vi "STB-Top.vi"() -> ()   [LabVIEW 2024]
doc: "This template is for the Queued Message Handler design pattern.\n\nThe Event Handling Loop generates messages based on user interface actions.\n\nThe Message Handling Loop processes messages generated by the Event Handling Loop, or by other messages. The messages are string values, so new messages can be added easily to the Message Cases case structure in the Message Handling Loop. Each message cluster can also provide an optional value for Message Data, which is a variant that can be converted to whatever message-specific data is required."
uses:
  e6b95c05-a4c0-4812-af30-7667d0d88226.vi
  <resource>/objmgr/daqmx.rc
  <vilib>/Utility/miscctls.llb/LVRectTypeDef.ctl
  <vilib>/Utility/TDMS File Viewer/NI_TDMS File Viewer.lvlib
panel:
  in  "Logging":bool
  out "IsLogging?":bool
  in  "Stop Button":bool
  in  "Save Settings":bool
  in  "Tab Control":T1(tab)
  in  "NI9205_Ch_3":bool
  in  "NI9205_Ch_2":bool
  in  "NI9205_Ch_1":bool
  in  "NI9205_Ch_0":bool
  in  "NI9219_Ch_3":bool
  in  "NI9219_Ch_2":bool
  in  "NI9219_Ch_1":bool
  in  "NI9219_Ch_0":bool
  in  "NI9219_Ch_2_Strain Gauge":bool
  in  "NI9219_Ch_1_Strain Gauge":bool
  in  "NI9219_Ch_0_Strain Gauge":bool
  in  "NI9219_Ch_0_Load Cell":bool
  out "Warnings & Messages":string
  out "NI9219_Channel 0-2 Chart":dynamicdata(graph)
  out "Temperature_6":dbl caption="Strain_2"
  out "Temperature_5":dbl caption="Strain_1"
  out "Temperature_4":dbl caption="Strain_0"
  out "NI9219_Channel 0Chart":dynamicdata(graph)
  out "Temperature_0":dbl caption="Force_0"
  out "NI9219_Channel 0-3 Chart":dynamicdata(graph)
  out "Temperature_3":dbl caption="Strain_3"
  out "Temperature_2":dbl caption="Strain_2"
  out "Temperature_1":dbl caption="Strain_1"
  out "Temperature_0":dbl caption="Strain_0"
  out "NI9205_Channel 0-3 Chart":dynamicdata(graph)
  out "Current_3":dbl caption="Voltage_3"
  out "Current_2":dbl caption="Voltage_2"
  out "Current_1":dbl caption="Voltage_1"
  out "Current_0":dbl caption="Voltage_0"
  out "Select File Path Analysis":path caption="Select File Path"
  in  "Offline Analysis":bool
  out "TDMS File Path":path
  # "These controls have associated \"Value Changed\" events configured in the Event Structure on the diagram.\n\nReplace them (and reconfigure the Event Structure) with the controls you need for your application."
  # "This template is for the Queued Message Handler design pattern.\n\nSee the block diagram for more information on how to use this template."
  # "Slot 1:NI 9219"
  # "Slot 1:NI 9219"
  # "Slot 2:NI 9219"
  # "NI 9205"
  # "Warnings & Messages"
  # "Picture"
  # "Channel 0-2"
  # "Channel 0"
  # "Channel 0-3"
  # "Channel 0-3"
  # "Analysis"
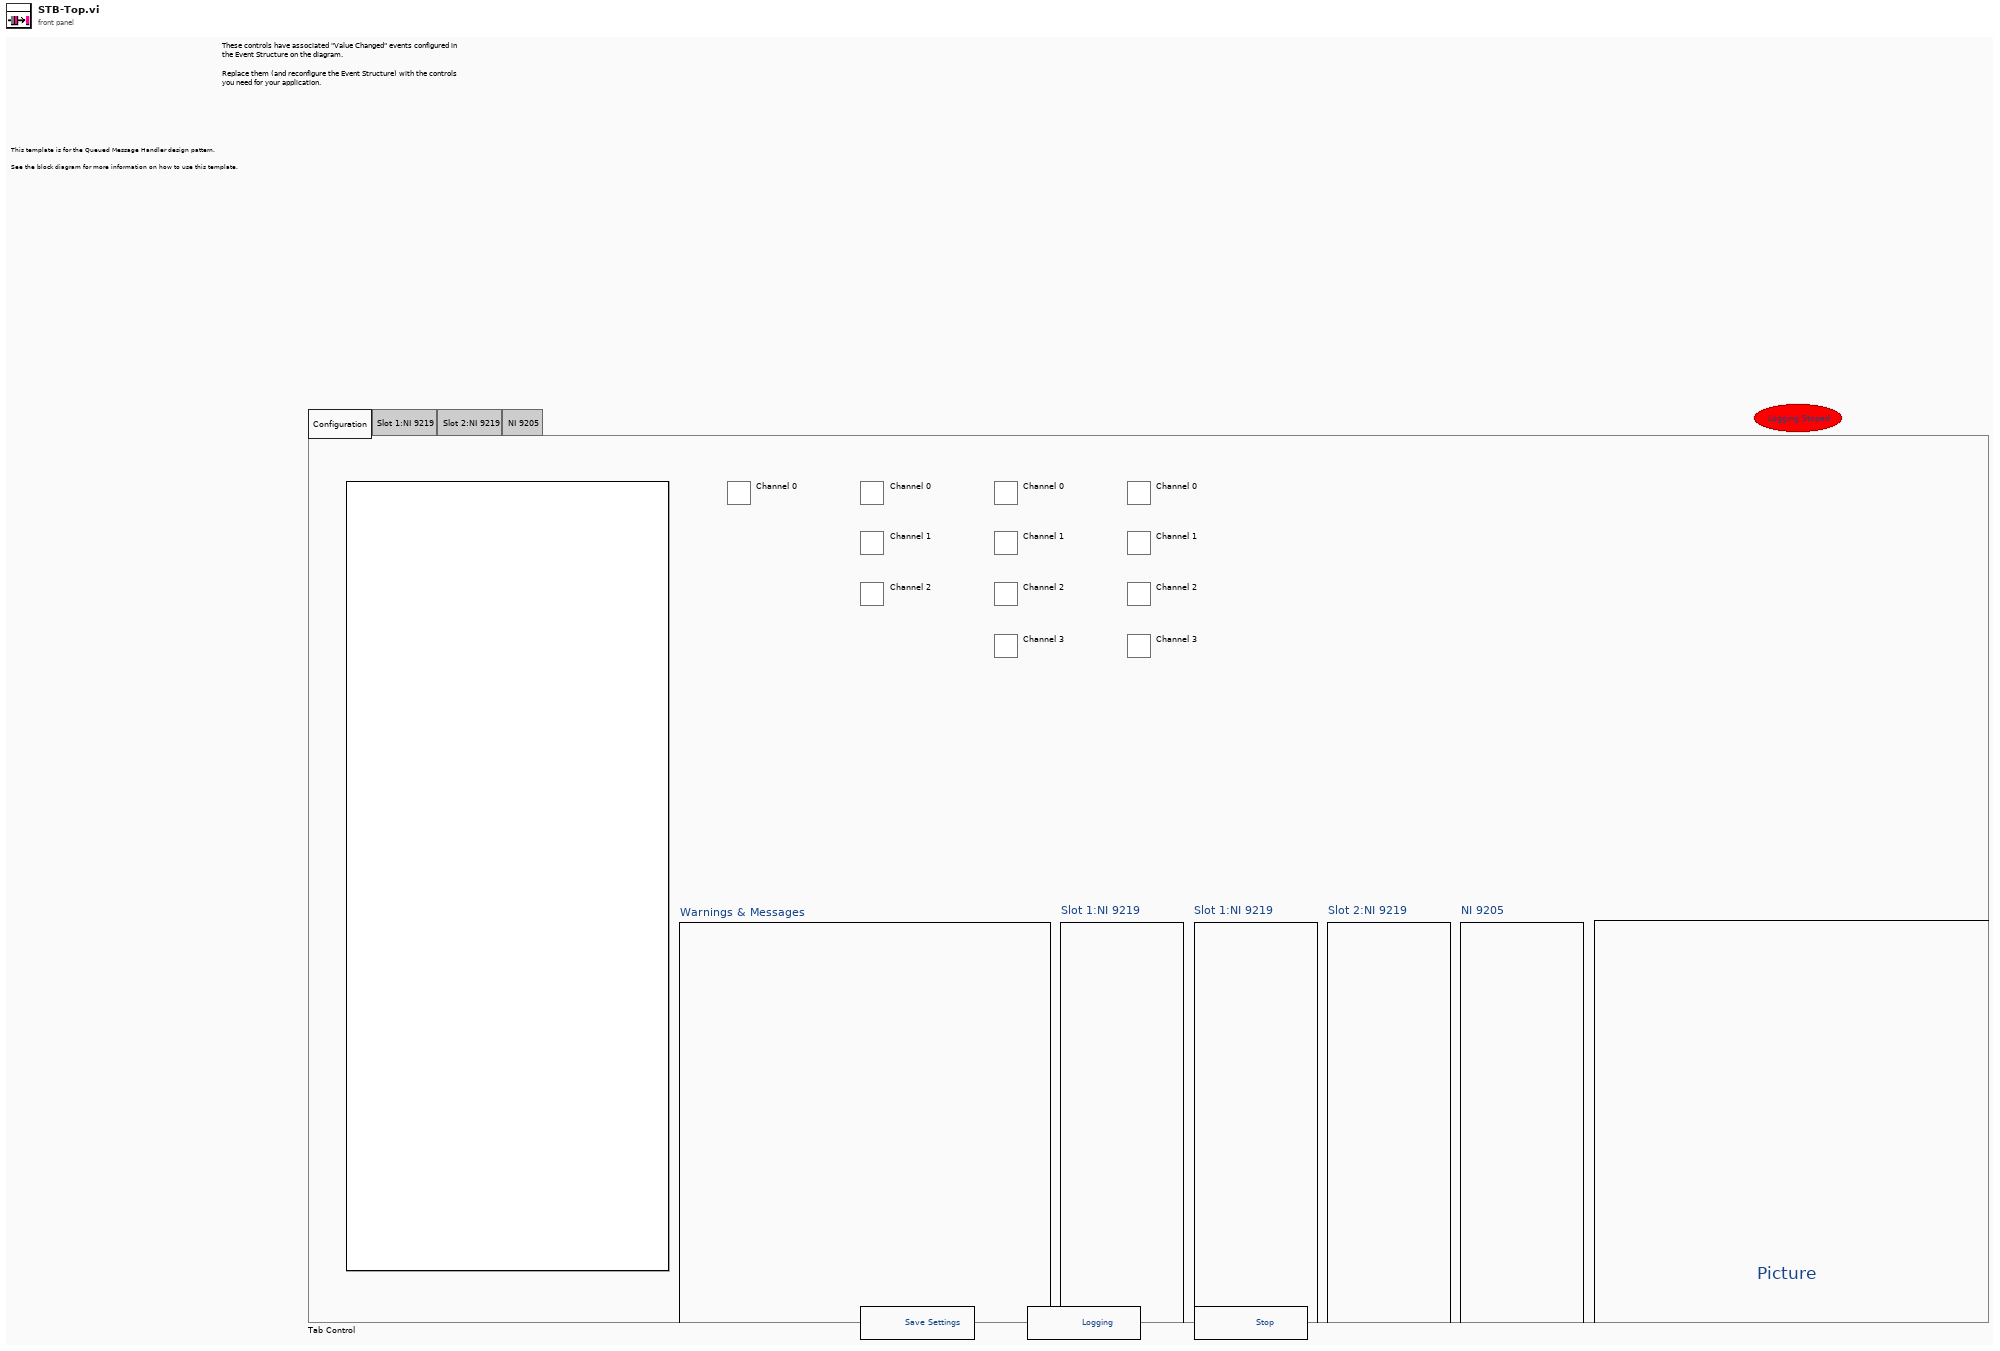
[diagram p1: front panel]
types:
  T1 = enum32{"Configuration", "Slot 1:NI 9219", "Slot 2:NI 9219", "NI 9205", "Offline Analysis"}
  T2 = typedef "LVRectTypeDef.ctl" = cluster{"Left":i16, "Top":i16, "Right":i16, "Bottom":i16}
  T3 = enum16{"open", "open or create", "create or replace", "create", "open (read-only)"}
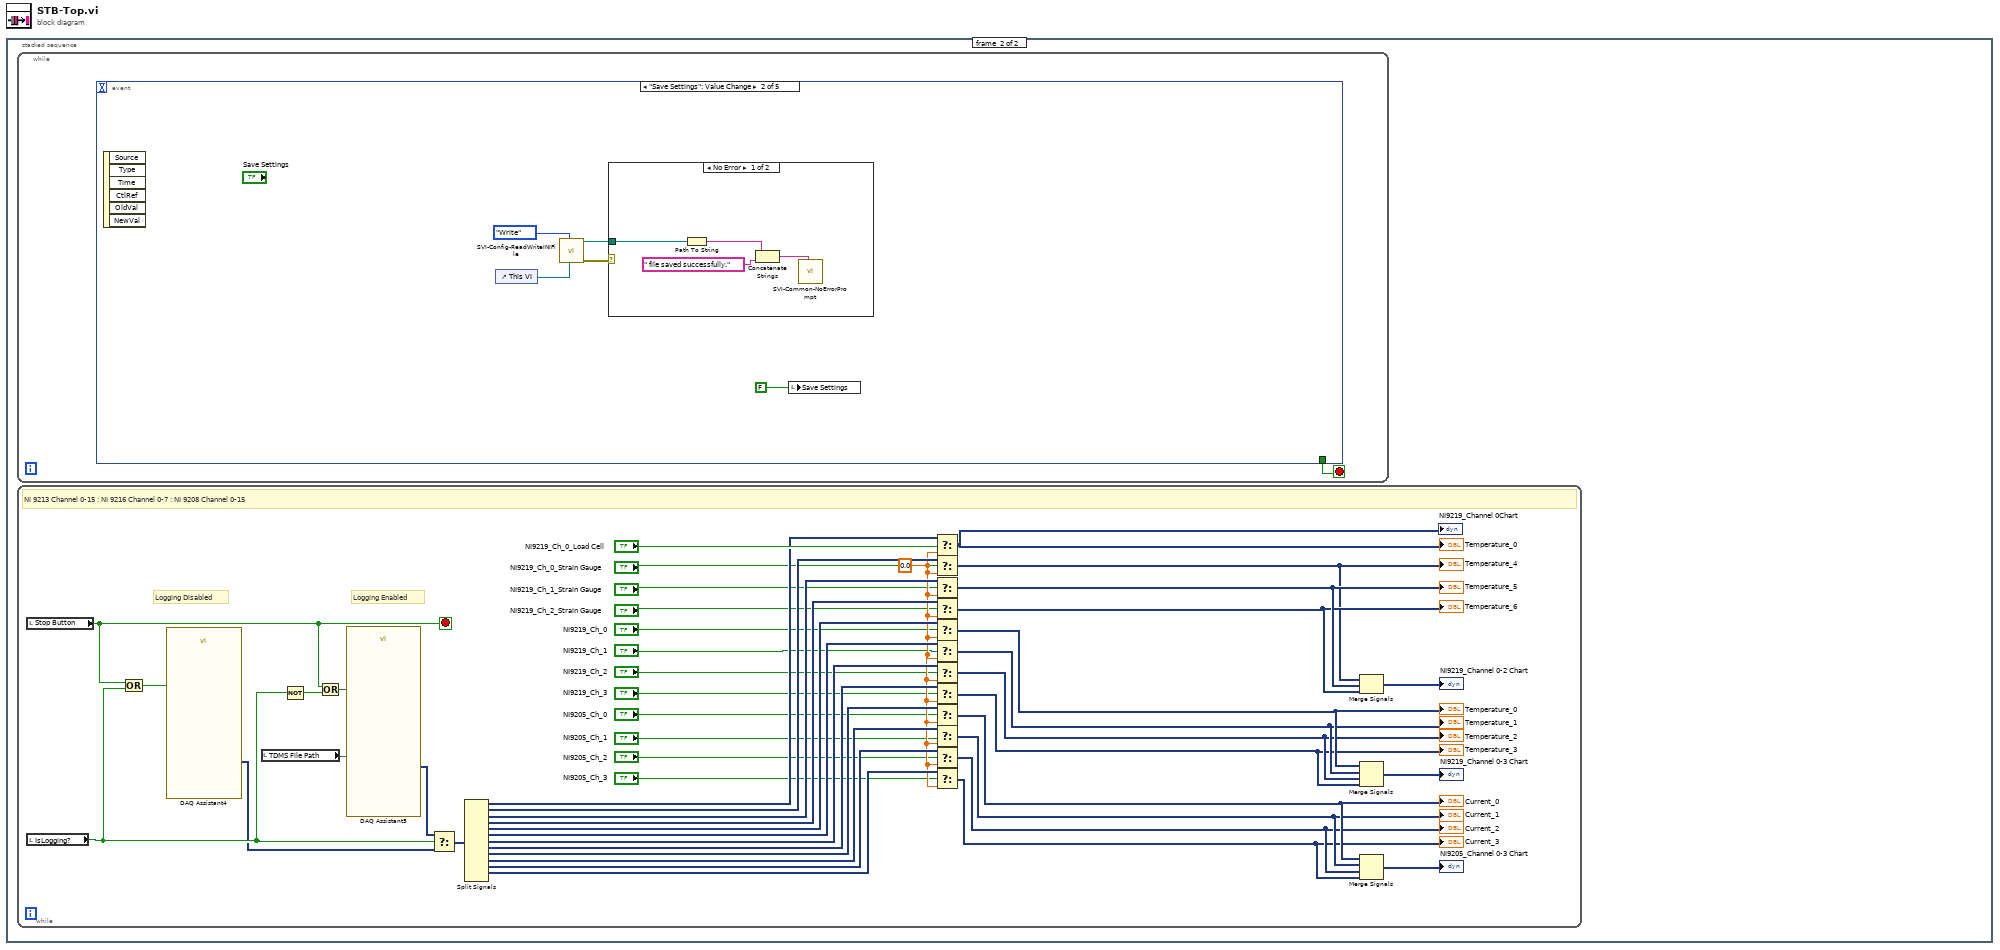
[diagram p0: block diagram]
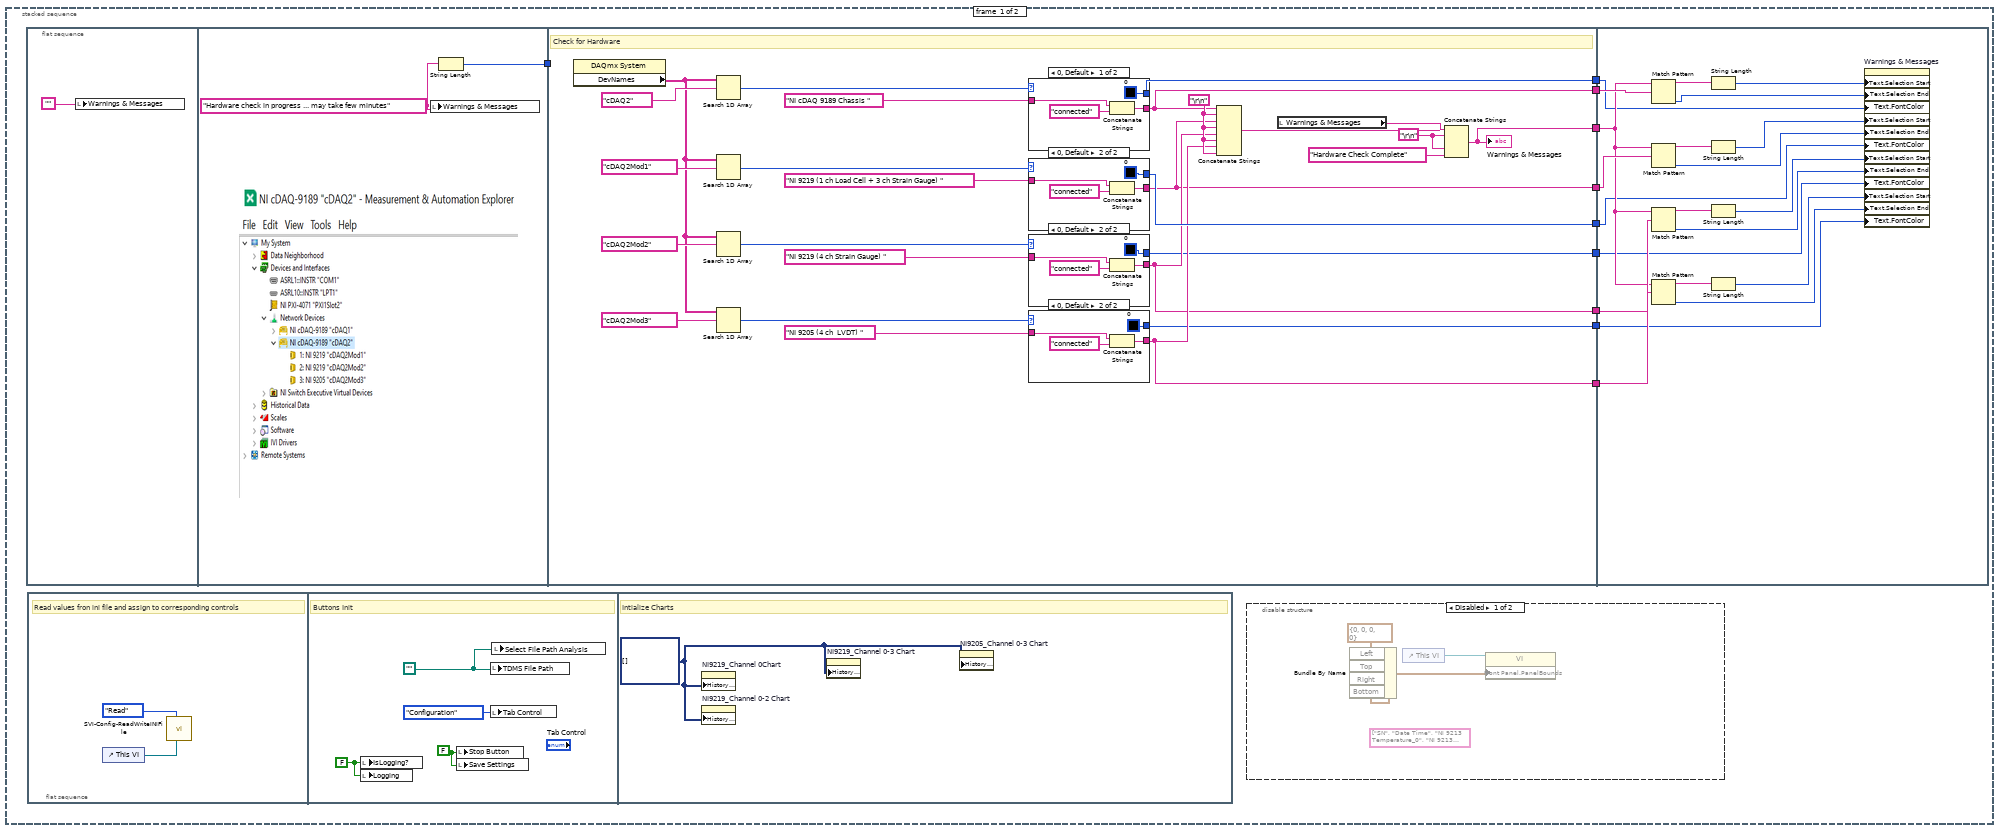
[diagram p2: hidden frame]
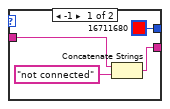
[diagram p4: hidden frame]
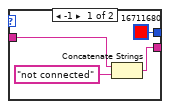
[diagram p5: hidden frame]
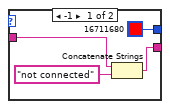
[diagram p6: hidden frame]
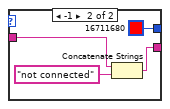
[diagram p7: hidden frame]
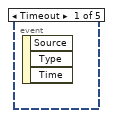
[diagram p8: hidden frame]
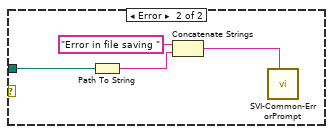
[diagram p9: hidden frame]
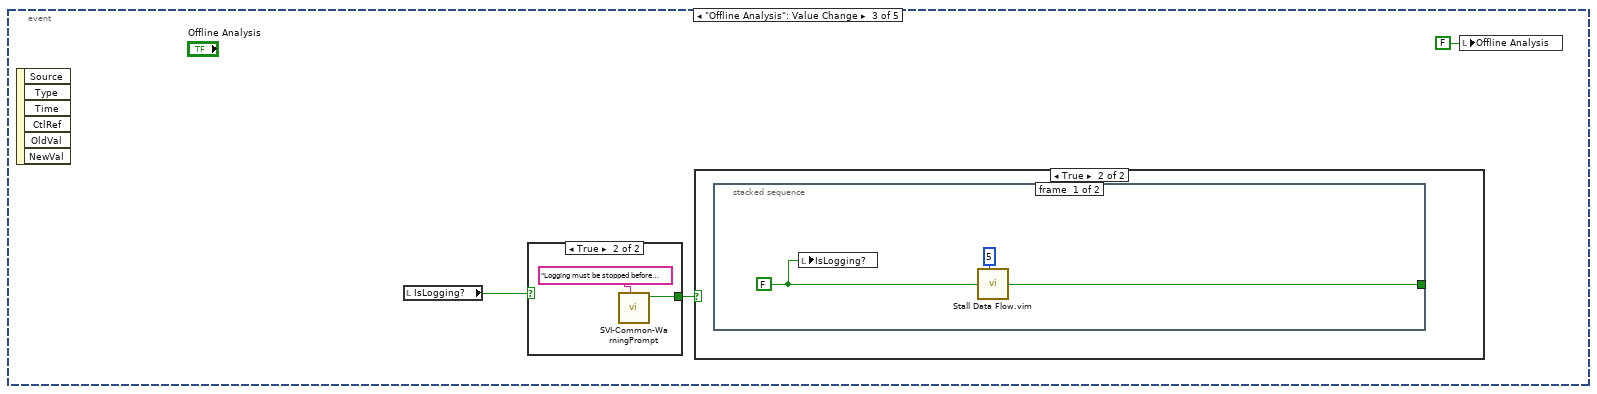
[diagram p10: hidden frame]
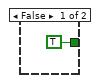
[diagram p11: hidden frame]
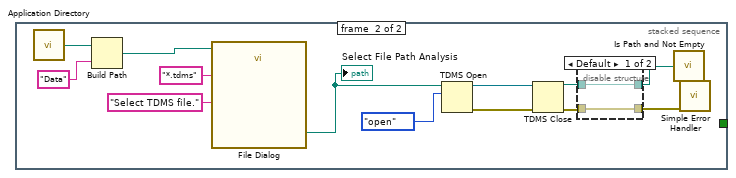
[diagram p13: hidden frame]
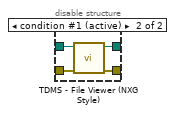
[diagram p14: hidden frame]
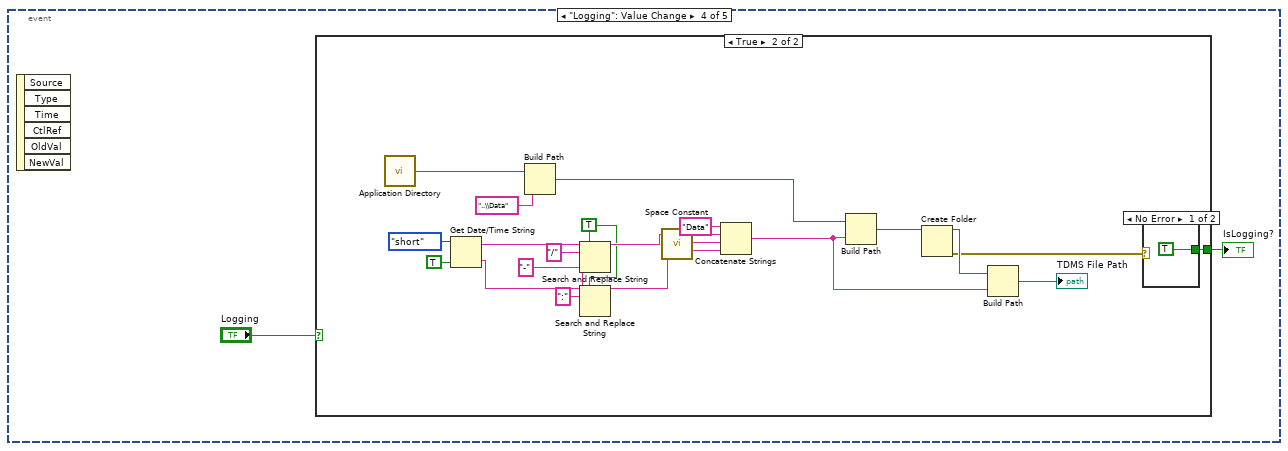
[diagram p15: hidden frame]
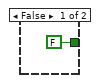
[diagram p16: hidden frame]
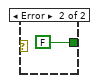
[diagram p17: hidden frame]
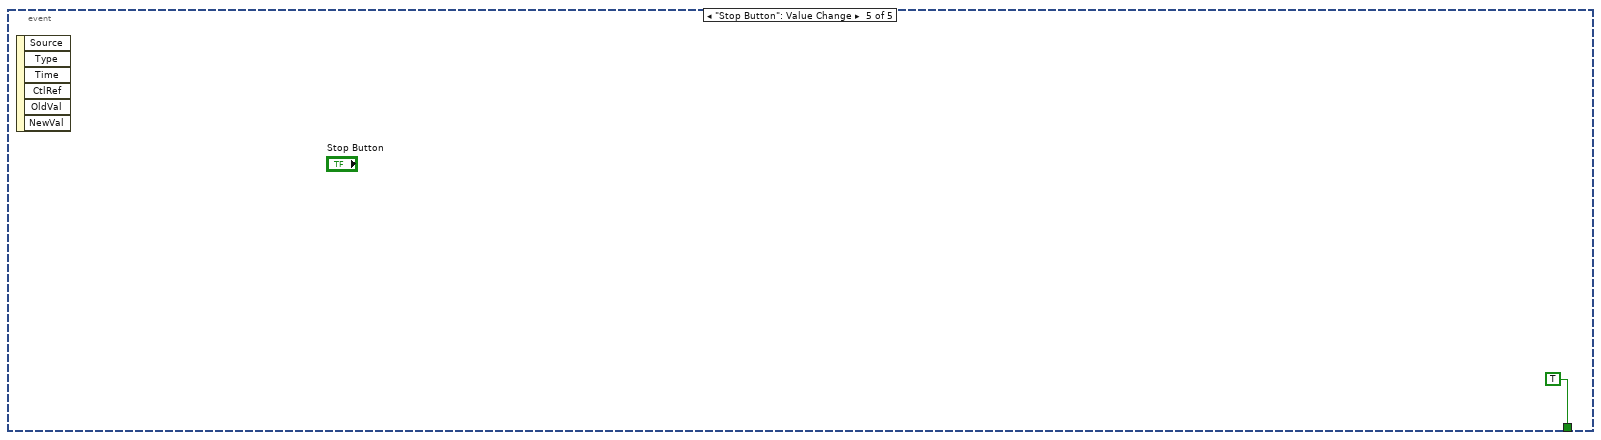
[diagram p18: hidden frame]
diagram:
  n1 = stacked-sequence {
    frame #0 {
      n2 = flat-sequence {
        tunnel: [w22] -> w10
        tunnel: w10 -> [_]
        tunnel: [w38] -> w9
        tunnel: [w37] -> w8
        tunnel: [w30] -> w7
        tunnel: [w29] -> w6
        tunnel: [w35] -> w5
        tunnel: [w34] -> w4
        tunnel: [w33] -> w3
        tunnel: [w32] -> w2
        tunnel: [w31] -> w1
        tunnel: w9 -> [w92]
        tunnel: w8 -> [w89]
        tunnel: w7 -> [w86]
        tunnel: w6 -> [w83]
        tunnel: w5 -> [w99]
        tunnel: w4 -> [w98]
        tunnel: w3 -> [w97]
        tunnel: w2 -> [w96]
        tunnel: w1 -> [w95]
        frame #0 {
          n3 = local write "Warnings & Messages"("") -> ()
        }
        frame #1 {
          w23 = "Hardware check in progress ... may take few minutes"
          n4 = local write "Warnings & Messages"(w23) -> ()
          n5 = String Length(string=w23) -> (length=w22:i32)
        }
        frame #2 {
          w40 = "\r\n"
          w47 = "\r\n"
          # "Check for Hardware"
          n6 = property class="DAQmx System"() -> ("DevNames"=w42:tag[])  [unwired: 2 in, 2 out]
          n7 = Search 1D Array(1D array=w42, element=tag "cDAQ2") -> (index of element=w28:i32)  [unwired: 1 in]
          n8 = Search 1D Array(1D array=w42, element=tag "cDAQ2Mod1") -> (index of element=w25:i32)  [unwired: 1 in]
          n9 = Search 1D Array(1D array=w42, element=tag "cDAQ2Mod2") -> (index of element=w24:i32)  [unwired: 1 in]
          n10 = Search 1D Array(1D array=w42, element=tag "cDAQ2Mod3") -> (index of element=w27:i32)  [unwired: 1 in]
          n11 = case shown="0, Default" w28 {
            tunnel: "NI cDAQ 9189 Chassis " -> [w78 w82]
            tunnel: [w76 w80] -> w32
            tunnel: [u32 0 ("Text.Text Colors:Text Color") u32 16711680 ("Text.Text Colors:Text Color")] -> w38
            frame 0, Default {
              n12 = Concatenate Strings(w78, "connected" ("string")) -> (w76:string)
            }
            frame -1 {
              n13 = Concatenate Strings(w82, "not connected" ("string")) -> (w80:string)
            }
          }
          n14 = case shown="0, Default" w25 {
            tunnel: "NI 9219 (1 ch Load Cell + 3 ch Strain Gauge) " -> [w70 w74]
            tunnel: [w68 w72] -> w33
            tunnel: [u32 16711680 ("Text.Text Colors:Text Color") u32 0 ("Text.Text Colors:Text Color")] -> w37
            frame -1 {
              n15 = Concatenate Strings(w70, "not connected" ("string")) -> (w68:string)
            }
            frame 0, Default {
              n16 = Concatenate Strings(w74, "connected" ("string")) -> (w72:string)
            }
          }
          n17 = case shown="0, Default" w24 {
            tunnel: "NI 9219 (4 ch Strain Gauge) " -> [w62 w66]
            tunnel: [w60 w64] -> w34
            tunnel: [u32 16711680 ("Text.Text Colors:Text Color") u32 0 ("Text.Text Colors:Text Color")] -> w30
            frame -1 {
              n18 = Concatenate Strings(w62, "not connected" ("string")) -> (w60:string)
            }
            frame 0, Default {
              n19 = Concatenate Strings(w66, "connected" ("string")) -> (w64:string)
            }
          }
          n20 = case shown="0, Default" w27 {
            tunnel: "NI 9205 (4 ch  LVDT) " -> [w54 w58]
            tunnel: [w52 w56] -> w35
            tunnel: [u32 16711680 ("Text.Text Colors:Text Color") u32 0 ("Text.Text Colors:Text Color")] -> w29
            frame -1 {
              n21 = Concatenate Strings(w54, "not connected" ("string")) -> (w52:string)
            }
            frame 0, Default {
              n22 = Concatenate Strings(w58, "connected" ("string")) -> (w56:string)
            }
          }
          n23 = Concatenate Strings(w32, w47, w33, w47, w34, w47, w35, w47) -> (w36:string)
          n24 = local read "Warnings & Messages"() -> (w41:string)
          n25 = Concatenate Strings(w41, w40, w36, w40, "Hardware Check Complete") -> (w31:string)
          "Warnings & Messages" <- w31
        }
        frame #3 {
          n26 = Match Pattern(string=w95, regular expression=w96) -> (before substring=w100:string, offset past match=w93:i32)  [unwired: 1 in, 2 out]
          n27 = Match Pattern(string=w95, regular expression=w97) -> (before substring=w101:string, offset past match=w90:i32)  [unwired: 1 in, 2 out]
          n28 = Match Pattern(string=w95, regular expression=w98) -> (before substring=w102:string, offset past match=w87:i32)  [unwired: 1 in, 2 out]
          n29 = Match Pattern(string=w95, regular expression=w99) -> (before substring=w103:string, offset past match=w84:i32)  [unwired: 1 in, 2 out]
          n30 = String Length(string=w100) -> (length=w94:i32)
          n31 = String Length(string=w101) -> (length=w91:i32)
          n32 = String Length(string=w102) -> (length=w88:i32)
          n33 = String Length(string=w103) -> (length=w85:i32)
          n34 = property on="Warnings & Messages" class="Str"("Text.Selection Start"=w94, "Text.Selection End"=w93, "Text.FontColor"=w92, "Text.Selection Start"=w91, "Text.Selection End"=w90, "Text.FontColor"=w89, "Text.Selection Start"=w88, "Text.Selection End"=w87, "Text.FontColor"=w86, "Text.Selection Start"=w85, "Text.Selection End"=w84, "Text.FontColor"=w83) -> ()  [unwired: 2 in, 2 out]
        }
      }
      n35 = flat-sequence {
        frame #0 {
          # "Read values fron ini file and assign to corresponding controls"
          n36 = control-ref of="This VI"() -> (w15:refnum<vi>)
          n37 = call "SVI-Config-ReadWriteINIFile.vi"("VI ref"=w15, "Mode"=enum16{"Read", "Write"}."Read") -> ()  [unwired: 8 in, 2 out]
        }
        frame #1 {
          w18 = path ""
          w16 = FALSE ("Stop Button 3")
          w19 = FALSE ("Logging")
          # "Buttons Init"
          n38 = local write "IsLogging?"(w16) -> ()
          n39 = local write "Logging"(w16) -> ()
          n40 = local write "Stop Button"(w19) -> ()
          n41 = local write "Save Settings"(w19) -> ()
          n42 = local write "TDMS File Path"(w18) -> ()
          n43 = local write "Tab Control"(T1."Configuration" ("Tab Control")) -> ()
          n44 = local write "Select File Path Analysis"(w18) -> ()
        }
        frame #2 {
          w20 = dynamicdata[] [] ("History Data")
          # "Intialize Charts"
          n45 = property on="NI9219_Channel 0Chart" class="WFChart (strict)"("History Data"=w20) -> ()  [unwired: 2 in, 2 out]
          n46 = property on="NI9219_Channel 0-2 Chart" class="WFChart (strict)"("History Data"=w20) -> ()  [unwired: 2 in, 2 out]
          n47 = property on="NI9219_Channel 0-3 Chart" class="WFChart (strict)"("History Data"=w20) -> ()  [unwired: 2 in, 2 out]
          n48 = property on="NI9205_Channel 0-3 Chart" class="WFChart (strict)"("History Data"=w20) -> ()  [unwired: 2 in, 2 out]
        }
      }
      n49 = disable-structure shown="Disabled" {
        frame Disabled {
          (unwired) string[] ["SN", "Date Time", "NI 9213 Temperature_0", "NI 9213 Temperature_1", "NI 9213 Temperature_2", "NI 9213 Temperature_3", "NI 9213 Temperature_4", "NI 9213 Temperature_5", "NI 9213 Temperature_6", "NI 9213 Temperature_7", "NI 9213 Temperature_8", "NI 9213 Temperature_9", "NI 9213 Temperature_10", "NI 9213 Temperature_11", "NI 9213 Temperature_12", "NI 9213 Temperature_13", "NI 9213 Temperature_14", "NI 9213 Temperature_15", "", "NI 9216 Temperature_0", "NI 9216 Temperature_1", "NI 9216 Temperature_2", "NI 9216 Temperature_3", "NI 9216 Temperature_4", "NI 9216 Temperature_5", "NI 9216 Temperature_6", "NI 9216 Temperature_7", "", "NI 9208 Current_0", "NI 9208 Current_1", "NI 9208 Current_2", "NI 9208 Current_3", "NI 9208 Current_4", "NI 9208 Current_5", "NI 9208 Current_6", "NI 9208 Current_7", "NI 9208 Current_8", "NI 9208 Current_9", "NI 9208 Current_10", "NI 9208 Current_11", "NI 9208 Current_12", "NI 9208 Current_13", "NI 9208 Current_14", "NI 9208 Current_15", "", "NI 9476 DigitalOut_0", "NI 9476 DigitalOut_1", "NI 9476 DigitalOut_2", "NI 9476 DigitalOut_3", "NI 9476 DigitalOut_4", "NI 9476 DigitalOut_5", "NI 9476 DigitalOut_6", "NI 9476 DigitalOut_7", "NI 9476 DigitalOut_8", "NI 9476 DigitalOut_9", "NI 9476 DigitalOut_10", "NI 9476 DigitalOut_11", "NI 9476 DigitalOut_12", "NI 9476 DigitalOut_13", "NI 9476 DigitalOut_14", "NI 9476 DigitalOut_15", "NI 9476 DigitalOut_16", "NI 9476 DigitalOut_17", "NI 9476 DigitalOut_18", "NI 9476 DigitalOut_19", "NI 9476 DigitalOut_20", "NI 9476 DigitalOut_21", "NI 9476 DigitalOut_22", "NI 9476 DigitalOut_23", "NI 9476 DigitalOut_24", "NI 9476 DigitalOut_25", "NI 9476 DigitalOut_26", "NI 9476 DigitalOut_27", "NI 9476 DigitalOut_28", "NI 9476 DigitalOut_29", "NI 9476 DigitalOut_30", "NI 9476 DigitalOut_31"] ("appended array")
          n50 = Bundle By Name(cluster=T2 {"Left"=0, "Top"=0, "Right"=0, "Bottom"=0} ("Front Panel Window:Panel Bounds")) -> (w12:T2)  [unwired: 4 in]
          n51 = control-ref of="This VI"() -> (w13:refnum<vi>)
          n52 = property class="VI"(reference=w13, "Front Panel.PanelBounds"=w12) -> ()  [unwired: 1 in, 2 out]
        }
        frame Enabled {
        }
      }
    }
    frame #1 {
      n53 = while {
        stop <- w104 stop-if-true
        n54 = event shown="[1] \"Save Settings\": Value Change" {
          selector: _ -> [_ _ _ _ _]
          dyn-events: _ -> [_ _ _ _ _]
          timeout: _ -> [_ _ _ _ _]
          tunnel: [_ _ _ _ TRUE] -> w104
          event Timeout {
            n55 = event-data() -> ()  [unwired: 1 in, 3 out]
          }
          event "Save Settings": Value Change {
            n56 = event-data() -> ()  [unwired: 1 in, 6 out]
            n57 = control-ref of="This VI"() -> (w109:refnum<vi>)
            n58 = call "SVI-Config-ReadWriteINIFile.vi"("VI ref"=w109, "Mode"=enum16{"Read", "Write"}."Write") -> ("error out"=w105:errorcluster, "Path"=w107:path)  [unwired: 8 in]
            n59 = case shown="No Error" w105 {
              tunnel: w107 -> [w112 w116]
              frame No Error {
                n60 = Path To String(path=w112) -> (string=w111:string)
                n61 = Concatenate Strings(w111, " file saved successfully." ("MsgIn")) -> (w110:string)
                n62 = call "SVI-Common-NoErrorPrompt.vi"("MsgIn"=w110) -> ()  [unwired: 11 in]
              }
              frame Error {
                n63 = Path To String(path=w116) -> (string=w114:string)
                n64 = Concatenate Strings("Error in file saving " ("string"), w114) -> (w115:string)
                n65 = call "SVI-Common-ErrorPrompt.vi"("MsgIn"=w115) -> ()  [unwired: 11 in]
              }
            }
            n66 = local write "Save Settings"(FALSE ("Save Settings Button")) -> ()
          }
          event "Offline Analysis": Value Change {
            n67 = event-data() -> ()  [unwired: 1 in, 6 out]
            n68 = local read "IsLogging?"() -> (w118:bool)
            n69 = case shown="True" w118 {
              tunnel: [TRUE ("Status") w122] -> w119
              frame False {
              }
              frame True {
                n70 = call "SVI-Common-WarningPrompt.vi"("MsgIn"="Logging must be stopped before analysis. Are you sure you want to stop logging?") -> ("Status"=w122:bool)  [unwired: 10 in]
              }
            }
            n71 = case shown="True" w119 {
              frame False {
              }
              frame True {
                n72 = stacked-sequence {
                  tunnel: [w125 _] -> _
                  frame #0 {
                    w124 = FALSE ("Stop Logging")
                    n73 = local write "IsLogging?"(w124) -> ()
                    n74 = call "Stall Data Flow.vim"("value in"=w124, "milliseconds to wait"=u32 5) -> ("value out"=w125:bool)  [unwired: 1 out]
                  }
                  frame #1 {
                    n75 = call <vilib>:"Application Directory.vi"() -> ("Application Directory"=w132:path)
                    n76 = Build Path(base path=w132, name or relative path="Data") -> (appended path=w130:path)
                    n77 = call "File Dialog"("start path"=w130, "prompt"="Select TDMS file.", "pattern (all files)"="*.tdms") -> ("selected path"=w127:path)  [unwired: 9 in, 3 out]
                    "Select File Path Analysis" <- w127
                    n78 = TDMS Open(10:T3."open" ("operation"), 11:w127) -> (0:w135:errorcluster, 3:w134:refnum<k34>)  [unwired: 5 in]
                    n79 = TDMS Close(8:w135, 11:w134) -> (0:w137:errorcluster, 3:w138:path)
                    n80 = disable-structure shown="Default" {
                      disable-tunnel: w137 -> [w141 w145]
                      disable-tunnel: w138 -> [w140 w144]
                      disable-tunnel: [w141 w143] -> w136
                      disable-tunnel: [w140 w142] -> w133
                      frame condition #0 {
                      }
                      frame condition #1 (active) {
                        n81 = call <vilib>:"TDMS - File Viewer (NXG Style).vi"("error in"=w145, "file in"=w144) -> ("error out"=w143:errorcluster, "file out"=w142:path)  [unwired: 8 in]
                      }
                    }
                    n82 = call <vilib>:"Is Path and Not Empty.vi"("path"=w133) -> ()  [unwired: 4 in, 1 out]
                    n83 = call <vilib>:"Simple Error Handler.vi"("error in (no error)"=w136) -> ()  [unwired: 4 in, 5 out]
                  }
                }
              }
            }
            n84 = local write "Offline Analysis"(FALSE ("Offline Analysis")) -> ()
          }
          event "Logging": Value Change {
            n85 = event-data() -> ()  [unwired: 1 in, 6 out]
            n86 = case shown="True" "Logging" {
              tunnel: [FALSE ("IsLogging?") w149] -> w146
              frame False {
              }
              frame True {
                w157 = TRUE ("replace all? (F)")
                w155 = "-" ("replace string (\"\")")
                n87 = call <vilib>:"Application Directory.vi"() -> ("Application Directory"=w164:path)
                n88 = Get Date/Time String(date format (0)=enum16{"short", "long", "abbreviated"}."short", want seconds? (F)=TRUE) -> (date string=w168:string, time string=w169:string)  [unwired: 1 in]
                n89 = Build Path(base path=w164, name or relative path="..\\Data") -> (appended path=w163:path)
                n90 = Search and Replace String(replace all?=w157, input string=w168, search string="/" ("substring (\"\")"), replace string=w155) -> (result string=w167:string)  [unwired: 4 in, 3 out]
                n91 = Search and Replace String(replace all?=w157, input string=w169, search string=":" ("replace string (\"\")"), replace string=w155) -> (result string=w165:string)  [unwired: 4 in, 3 out]
                n92 = call <vilib>:"Space Constant.vi"() -> ("String"=w166:string)
                n93 = Concatenate Strings("Data" ("string"), w167, w166, w165) -> (w161:string)
                n94 = Build Path(base path=w163, name or relative path=w161) -> (appended path=w162:path)
                n95 = Create Folder(path (use dialog)=w162) -> (created path=w151:path, error out=w150:errorcluster)  [unwired: 2 in, 1 out]
                n96 = Build Path(base path=w151, name or relative path=w161) -> (appended path=→"TDMS File Path":path)
                n97 = case shown="No Error" w150 {
                  tunnel: [TRUE ("IsLogging?") FALSE ("IsLogging?")] -> w149
                  frame No Error {
                  }
                  frame Error {
                  }
                }
              }
            }
            "IsLogging?" <- w146
          }
          event "Stop Button": Value Change {
            n98 = event-data() -> ()  [unwired: 1 in, 6 out]
          }
        }
      }
      n99 = while {
        stop <- w221 stop-if-true
        w204 = 0.0
        # "Logging Disabled"
        # "Logging Enabled"
        # "NI 9213 Channel 0-15 : NI 9216 Channel 0-7 : NI 9208 Channel 0-15"
        n100 = local read "Stop Button"() -> (w221:bool)
        n101 = local read "IsLogging?"() -> (w203:bool)
        n102 = Or(x=w221, y=w203) -> (x .or. y?=w201:bool)
        n103 = call "DAQ Assistant4"("stop (F)"=w201) -> ("data"=w200:dynamicdata)  [unwired: 15 in, 3 out]
        n104 = local read "TDMS File Path"() -> (w198:path)
        n105 = Not(x=w203) -> (.not. x?=w202:bool)
        n106 = Or(x=w221, y=w202) -> (x .or. y?=w199:bool)
        n107 = call "DAQ Assistant5"("stop (F)"=w199, "file path"=w198) -> ("data"=w197:dynamicdata)  [unwired: 14 in, 3 out]
        n108 = Select(t=w197, s=w203, f=w200) -> (s? t:f=w220:dynamicdata)
        n109 = Split Signals(w220) -> (w216:dynamicdata, w215:dynamicdata, w214:dynamicdata, w213:dynamicdata, w212:dynamicdata, w211:dynamicdata, w210:dynamicdata, w209:dynamicdata, w208:dynamicdata, w207:dynamicdata, w206:dynamicdata, w205:dynamicdata)  [unwired: 13 in, 1 out]
        n110 = Select(t=w216, s="NI9219_Ch_0_Load Cell", f=w204) -> (s? t:f=→"Temperature_0" →"NI9219_Channel 0Chart":dynamicdata)
        n111 = Select(t=w215, s="NI9219_Ch_0_Strain Gauge", f=w204) -> (s? t:f=w173:dynamicdata)
        "Temperature_4" <- w173
        n112 = Select(t=w214, s="NI9219_Ch_1_Strain Gauge", f=w204) -> (s? t:f=w192:dynamicdata)
        "Temperature_5" <- w192
        n113 = Select(t=w213, s="NI9219_Ch_2_Strain Gauge", f=w204) -> (s? t:f=w191:dynamicdata)
        "Temperature_6" <- w191
        n114 = Select(t=w212, s="NI9219_Ch_0", f=w204) -> (s? t:f=w185:dynamicdata)
        "Temperature_0" <- w185
        n115 = Select(t=w211, s="NI9219_Ch_1", f=w204) -> (s? t:f=w184:dynamicdata)
        "Temperature_1" <- w184
        n116 = Select(t=w210, s="NI9219_Ch_2", f=w204) -> (s? t:f=w183:dynamicdata)
        "Temperature_2" <- w183
        n117 = Select(t=w209, s="NI9219_Ch_3", f=w204) -> (s? t:f=w182:dynamicdata)
        "Temperature_3" <- w182
        n118 = Select(t=w208, s="NI9205_Ch_0", f=w204) -> (s? t:f=w177:dynamicdata)
        "Current_0" <- w177
        n119 = Select(t=w207, s="NI9205_Ch_1", f=w204) -> (s? t:f=w176:dynamicdata)
        "Current_1" <- w176
        n120 = Select(t=w206, s="NI9205_Ch_2", f=w204) -> (s? t:f=w175:dynamicdata)
        "Current_2" <- w175
        n121 = Select(t=w205, s="NI9205_Ch_3", f=w204) -> (s? t:f=w174:dynamicdata)
        "Current_3" <- w174
        n122 = Merge Signals(w173, w192, w191) -> (→"NI9219_Channel 0-2 Chart":dynamicdata)
        n123 = Merge Signals(w185, w184, w183, w182) -> (→"NI9219_Channel 0-3 Chart":dynamicdata)
        n124 = Merge Signals(w177, w176, w175, w174) -> (→"NI9205_Channel 0-3 Chart":dynamicdata)
      }
    }
  }
